vi "get countries in aggregate.vi"(9 "countries":string[](array[string]), 10 "aggregate name":string, 11 "Refnum in":T1) -> (2 "country indexes":i32[](array[numeric]), 3 "Refnum out":T1)   [LabVIEW 2019]
uses:
  <vilib>/Utility/config.llb/Config Data RefNum.ctl
  <vilib>/Utility/config.llb/Read Key (String).vi
  <vilib>/Utility/config.llb/NI_LVConfig.lvlib
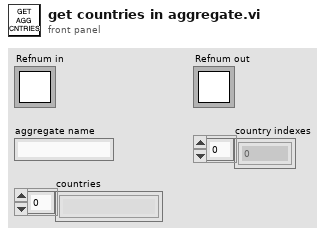
[diagram p1: front panel]
types:
  T1 = typedef "NI_LVConfig.lvlib/Config Data RefNum.ctl" = refnum<k1>
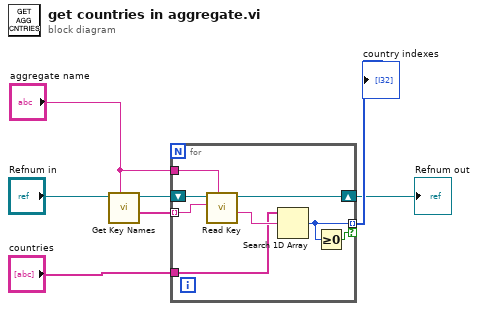
[diagram p0: block diagram]
diagram:
  n1 = call <vilib>:"Get Key Names.vi"("section"="aggregate name", "refnum"="Refnum in") -> ("key names"=w2:string[], "refnum out"=w1:T1)  [unwired: 6 in, 2 out]
  n2 = for {
    tunnel: w2 -> [w13] mode=indexing
    shift-right: [w14] -> w4
    shift-left: w1 -> [w15]
    tunnel: [w9] -> w5 mode=indexing if=w8
    tunnel: "aggregate name" -> [w12]
    tunnel: "countries" -> [w10]
    n3 = call-poly <vilib>:"Read Key.vi"("section"=w12, "key"=w13, "refnum"=w15) -> ("value"=w11:string, "refnum out"=w14:T1)  [unwired: 5 in, 2 out]
    n4 = Search 1D Array(1D array=w10, element=w11) -> (index of element=w9:i32)  [unwired: 1 in]
    n5 = Greater Or Equal To 0?(x=w9) -> (x >= 0?=w8:bool)
  }
  "country indexes" <- w5
  "Refnum out" <- w4
